vi "ZhiYuan ZDS Series for TCP Edge Triggered Acquisition.vi"() -> ()   [LabVIEW 2015]
doc: "This example shows how to configure the oscilloscope to perform an edge-triggered waveform acquisition."
uses:
  ZhiYuan ZDS Series for TCP.lvlib
  Public/Data/Read Waveform (Single).vi
panel:
  in  "Probe":i32(ring)=12 items=["0.001", "0.002", "0.005", "0.01", "0.02", "0.05", "0.1", "0.2", "0.5", "1", "2", "5", "10", "20", "50", "100", "200", "500", "1000"]
  in  "Edge Type":i32(ring) items=["Positive", "Negative", "Either"]
  in  "Scale(H)":T1(ring)=enum."50us"
  in  "Vertical Offset":dbl
  in  "Vertical Scale":dbl=1.0
  in  "Trigger Level":dbl=5.0
  in  "Vertical Coupling":i32(ring)=1 items=["AC", "DC", "GND"]
  in  "Offset (H)":dbl
  in  "Channel":i32(ring)=1 items=["Channel 1"=1, "Channel 2"=2, "Channel 3"=3, "Channel 4"=4]
  out "Waveform Data":dbl[](graph)
  in  "VISA resource name":refnum<visa-resource-name>
  # "(c) 2012 National Instruments.  ALL RIGHTS RESERVED."
  # "Vertical"
  # "Horizontal"
  # "Trigger"
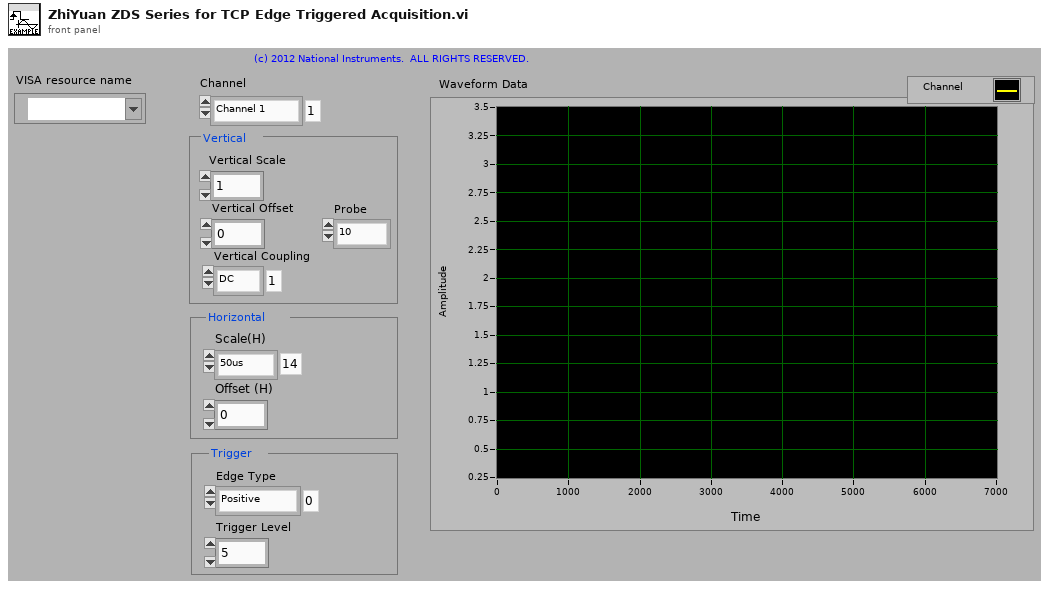
[diagram p1: front panel]
types:
  T1 = enum16{"1ns", "2ns", "5ns", "10ns", "20ns", "50ns", "100ns", "200ns", "500ns", "1us", "2us", "5us", "10us", "20us", "50us", "100us", "200us", "500us", "1ms", "2ms", "5ms", "10ms", "20ms", "50ms", "100ms", "200ms", "500ms", "1s", "2s", "5s", "10s", "20s", "50s", "100s"}
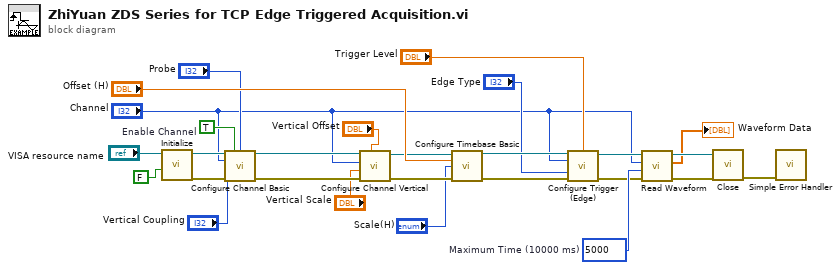
[diagram p0: block diagram]
diagram:
  w17 = TRUE  # Enable Channel
  w19 = u32 5000  # Maximum Time (10000 ms)
  n1 = call "Initialize.vi"("Reset (True)"=FALSE, "VISA resource name"="VISA resource name") -> ("error out"=w24:errorcluster, "VISA resource name out"=w25:refnum<visa-resource-name>)  [unwired: 8 in]
  n2 = call "Configure Channel Basic.vi"("VISA resource name"=w25, "Enable Channel (F: Disable)"=w17, "Probe"="Probe", "Channel (1: Channel 1)"="Channel", "Coupling Mode (1: DC)"="Vertical Coupling", "error in (no error)"=w24) -> ("VISA resource name out"=w11:refnum<visa-resource-name>, "error out"=w10:errorcluster)  [unwired: 8 in]
  n3 = call "Configure Channel Vertical.vi"("Offset (0)"="Vertical Offset", "error in (no error)"=w10, "Scale (1)"="Vertical Scale", "Channel (1: Channel 1)"="Channel", "VISA resource name"=w11) -> ("error out"=w8:errorcluster, "VISA resource name out"=w9:refnum<visa-resource-name>)  [unwired: 5 in]
  n4 = call "Configure Timebase Basic.vi"("VISA resource name"=w9, "Offset (0)"="Offset (H)", "Scale"="Scale(H)", "error in (no error)"=w8) -> ("VISA resource name out"=w14:refnum<visa-resource-name>, "error out"=w13:errorcluster)  [unwired: 10 in]
  n5 = call "Configure Trigger (Edge).vi"("VISA resource name"=w14, "Trigger Level (0)"="Trigger Level", "Source (1: Channel 1)"="Channel", "Edge Type (0: Positive)"="Edge Type", "error in (no error)"=w13) -> ("VISA resource name out"=w20:refnum<visa-resource-name>, "error out"=w18:errorcluster)  [unwired: 9 in]
  n6 = call-poly "Read Waveform.vi"("error in (no error)"=w18, "Maximum Time (5000 ms)"=w19, "Channel (1: Channel 1)"="Channel", "VISA resource name"=w20) -> ("error out"=w21:errorcluster, "Waveform Data"=→"Waveform Data":dbl[], "VISA resource name out"=w23:refnum<visa-resource-name>)  [unwired: 5 in]
  n7 = call "Close.vi"("error in (no error)"=w21, "VISA resource name"=w23) -> ("error out"=w27:errorcluster)  [unwired: 9 in]
  n8 = call <vilib>:"Simple Error Handler.vi"("error in (no error)"=w27) -> ()  [unwired: 4 in, 5 out]
